vi "Plotter.vi"(8 "error in (no error)":errorcluster, 11 "Plot_waveform in":refnum<class "Plot_waveform.lvclass">) -> (0 "error out":errorcluster, 2 "output waveform":waveform(dbl), 3 "Plot_waveform out":refnum<class "Plot_waveform.lvclass">)   [LabVIEW 2019, in "Plot_waveform.lvclass"]
uses:
  Plot_waveform.lvclass
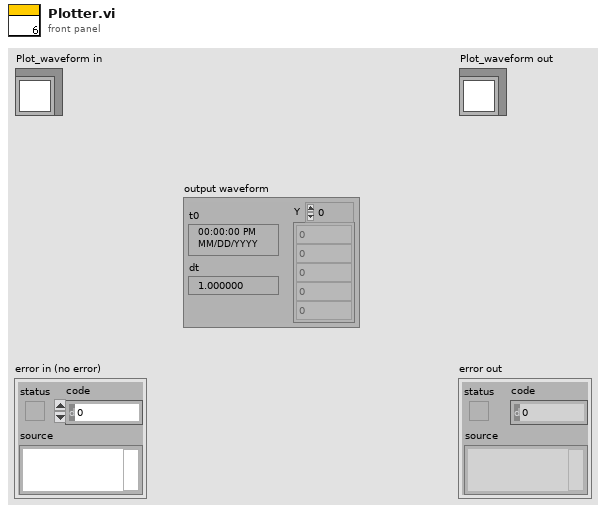
[diagram p1: front panel]
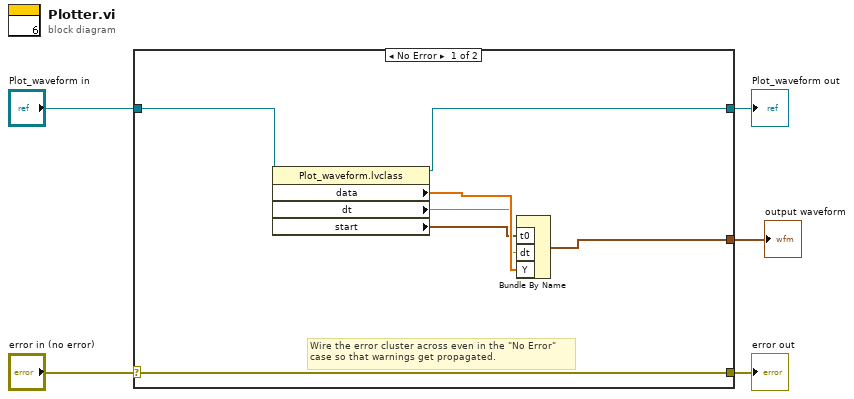
[diagram p0: block diagram]
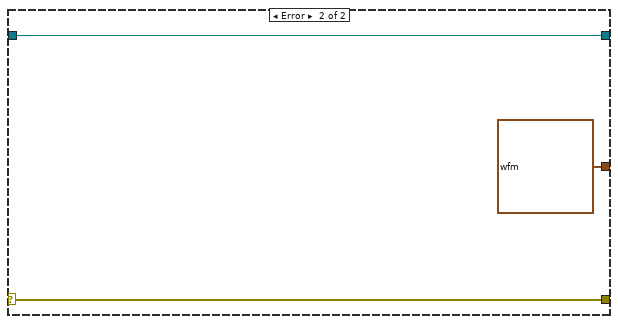
[diagram p2: hidden frame]
diagram:
  n1 = case shown="No Error" "error in (no error)" {
    selector: "error in (no error)" -> [w12 w15]
    tunnel: [w12 w15] -> w4
    tunnel: [w10 w14] -> w2
    tunnel: "Plot_waveform in" -> [w11 w14]
    tunnel: [w6 waveform(dbl) {"t0"=timestamp(0 s since 1904-01-01), "dt"=1.0, "Y"=[]}] -> w1
    frame No Error {
      # "Wire the error cluster across even in the \"No Error\"\ncase so that warnings get propagated."
      n2 = property class="Plot_waveform.lvclass"(reference=w11) -> (reference out=w10:refnum<class "Plot_waveform.lvclass">, "data"=w9:dbl[], "dt"=w8:dbl, "start"=w7:timestamp)  [unwired: 1 in, 1 out]
      n3 = Bundle By Name("t0"=w7, "dt"=w8, "Y"=w9) -> (w6:waveform(dbl))  [unwired: 1 in]
    }
    frame Error {
    }
  }
  "error out" <- w4
  "Plot_waveform out" <- w2
  "output waveform" <- w1
